vi "PArticle analysis.vi"() -> ()   [LabVIEW 2025]
uses:
  <vilib>/vision/NI_Vision_Development_Module.lvlib
panel:
  in  "White with color":bool
  out "Fail 2?":bool
  out "Fail 1?":bool
  out "Particle Reports (Pixels) 2":T1(array[cluster]) {"Orientation" format="%.2f"; "Dimensions"."Height" format="%.2f"; "Dimensions"."Width" format="%.2f"; "Center of Mass"."Y" format="%.2f"; "Center of Mass"."X" format="%.2f"; "Bounding Rect"."Bottom" format="%.2f"; "Bounding Rect"."Right" format="%.2f"; "Bounding Rect"."Top" format="%.2f"; "Bounding Rect"."Left" format="%.2f"; "Number of Holes" format="%.2f"; "Area" format="%.2f"}
  out "Particle Reports (Pixels)":T1(array[cluster]) {"Orientation" format="%.2f"; "Dimensions"."Height" format="%.2f"; "Dimensions"."Width" format="%.2f"; "Center of Mass"."Y" format="%.2f"; "Center of Mass"."X" format="%.2f"; "Bounding Rect"."Bottom" format="%.2f"; "Bounding Rect"."Right" format="%.2f"; "Bounding Rect"."Top" format="%.2f"; "Bounding Rect"."Left" format="%.2f"; "Number of Holes" format="%.2f"; "Area" format="%.2f"}
  out "Image 3":T2(plugin-control)
  out "Image 2":T2(plugin-control)
  out "Number of Particles 2":i32
  out "Number of Particles":i32
  out "Histogram Report 2":T3 {"Standard  Variation" format="%.2f"; "Mean Value" format="%.2f"; "Interval Width" format="%.2f"; "Starting Value" format="%.2f"; "Maximal Value" format="%.2f"; "Minimal Value" format="%.2f"}
  out "Image":T2(plugin-control)
  out "Histogram Report":T3 {"Standard  Variation" format="%.2f"; "Mean Value" format="%.2f"; "Interval Width" format="%.2f"; "Starting Value" format="%.2f"; "Maximal Value" format="%.2f"; "Minimal Value" format="%.2f"}
  in  "Interval Range":cluster{"Minimum":sgl, "Maximum":sgl} {"Maximum" format="%.2f"; "Minimum" format="%.2f"}
  # "1872"
  # "28883"
  # "31424"
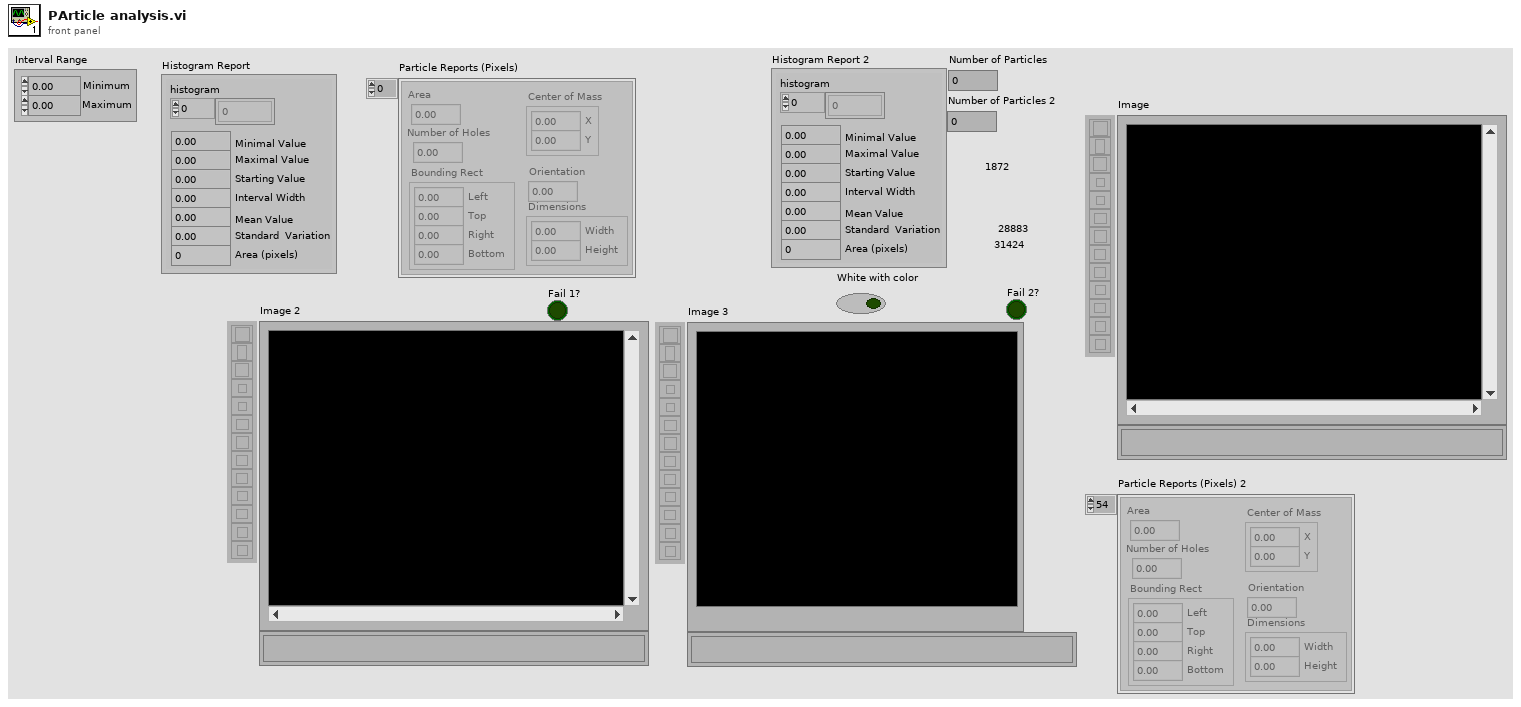
[diagram p1: front panel]
types:
  T1 = cluster{"Area":dbl, "Number of Holes":dbl, "Bounding Rect":cluster{"Left":dbl, "Top":dbl, "Right":dbl, "Bottom":dbl}, "Center of Mass":cluster{"X":dbl, "Y":dbl}, "Orientation":dbl, "Dimensions":cluster{"Width":dbl, "Height":dbl}}[]
  T2 = typedef "IMAQ Image.ctl" = refnum<image>
  T3 = cluster{"histogram":u32[], "Minimal Value":sgl, "Maximal Value":sgl, "Starting Value":sgl, "Interval Width":sgl, "Mean Value":sgl, "Standard  Variation":sgl, "Area (pixels)":i32}
  T4 = typedef "Image Type" = u32
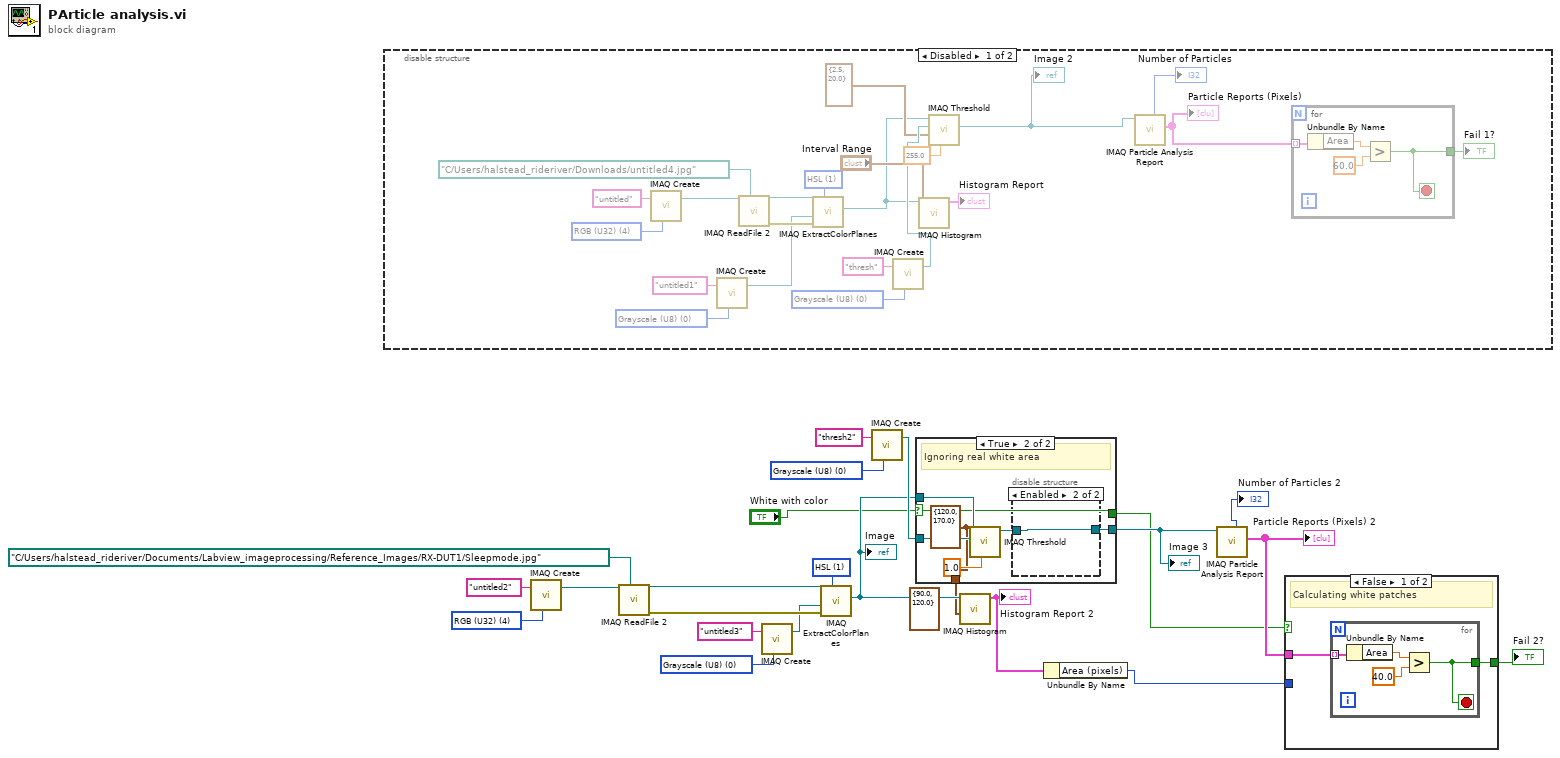
[diagram p0: block diagram]
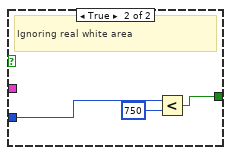
[diagram p3: hidden frame]
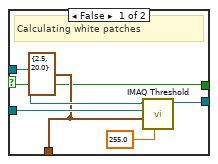
[diagram p4: hidden frame]
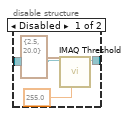
[diagram p5: hidden frame]
diagram:
  w13 = T4 0 items=["Grayscale (U8)", "Grayscale (I16)", "Grayscale (SGL)", "Complex (CSG)", "RGB (U32)", "HSL (U32)", "RGB (U64)", "Grayscale (U16)"] ("Image Type")
  (unwired) cluster{"Minimum":sgl, "Maximum":sgl} {"Minimum"=90.0, "Maximum"=120.0} ("Interval Range")
  w22 = u16 1 items=["RGB", "HSL", "HSV", "HSI"] ("Color Mode")
  w17 = T4 0 items=["Grayscale (U8)", "Grayscale (I16)", "Grayscale (SGL)", "Complex (CSG)", "RGB (U32)", "HSL (U32)", "RGB (U64)", "Grayscale (U16)"] ("Image Type")
  w16 = T4 4 items=["Grayscale (U8)", "Grayscale (I16)", "Grayscale (SGL)", "Complex (CSG)", "RGB (U32)", "HSL (U32)", "RGB (U64)", "Grayscale (U16)"] ("Image Type")
  n1 = disable-structure shown="Disabled" {
    frame Disabled {
      w33 = T4 0 items=["Grayscale (U8)", "Grayscale (I16)", "Grayscale (SGL)", "Complex (CSG)", "RGB (U32)", "HSL (U32)", "RGB (U64)", "Grayscale (U16)"] ("Image Type")
      w38 = u16 1 items=["RGB", "HSL", "HSV", "HSI"] ("Color Mode")
      w43 = T4 0 items=["Grayscale (U8)", "Grayscale (I16)", "Grayscale (SGL)", "Complex (CSG)", "RGB (U32)", "HSL (U32)", "RGB (U64)", "Grayscale (U16)"] ("Image Type")
      w44 = T4 4 items=["Grayscale (U8)", "Grayscale (I16)", "Grayscale (SGL)", "Complex (CSG)", "RGB (U32)", "HSL (U32)", "RGB (U64)", "Grayscale (U16)"] ("Image Type")
      n2 = call "IMAQ Create"("Image Name"="untitled", "Image Type"=w44) -> ("New Image"=w41:T2)  [unwired: 3 in, 1 out]
      n3 = call "IMAQ Create"("Image Name"="untitled1", "Image Type"=w43) -> ("New Image"=w30:T2)  [unwired: 3 in, 1 out]
      n4 = call "IMAQ ReadFile 2"("File Path"=path "C:/Users/halstead_rideriver/Downloads/untitled4.jpg", "Image"=w41) -> ("error out"=w39:errorcluster, "Image Out"=w37:T2)  [unwired: 5 in, 3 out]
      n5 = call "IMAQ ExtractColorPlanes"("Color Mode"=w38, "error in (no error)"=w39, "Green or Sat Plane"=w30, "Image Src"=w37) -> ("Green or Sat Plane out"=w29:T2)  [unwired: 4 in, 3 out]
      n6 = call "IMAQ Create"("Image Name"="thresh", "Image Type"=w33) -> ("New Image"=w32:T2)  [unwired: 3 in, 1 out]
      n7 = call "IMAQ Histogram"("Interval Range"="Interval Range", "Image"=w29) -> ("Histogram Report"=→"Histogram Report":T3)  [unwired: 8 in, 1 out]
      n8 = call "IMAQ Threshold"("Replace Value"=sgl 255.0, "Range"=cluster{"Lower value":sgl, "Upper value":sgl} {"Lower value"=2.5, "Upper value"=20.0}, "Image Dst"=w32, "Image Src"=w29) -> ("Image Dst Out"=w27:T2)  [unwired: 6 in, 1 out]
      "Image 2" <- w27
      n9 = call "IMAQ Particle Analysis Report"("Image"=w27) -> ("Particle Reports (Pixels)"=w25:T1, "Number of Particles"=→"Number of Particles":i32)  [unwired: 5 in, 4 out]
      "Particle Reports (Pixels)" <- w25
      n10 = for {
        tunnel: w25 -> [w49] mode=indexing
        tunnel: [w46] -> w26
        stop <- w46 stop-if-true
        n11 = Unbundle By Name(w49) -> ("Area"=w48:dbl)
        n12 = Greater?(x=w48, y=60.0) -> (0:w46:bool)
      }
      "Fail 1?" <- w26
    }
    frame Enabled {
    }
  }
  n13 = call "IMAQ Create"("Image Name"="untitled2", "Image Type"=w16) -> ("New Image"=w19:T2)  [unwired: 3 in, 1 out]
  n14 = call "IMAQ ReadFile 2"("File Path"=path "C:/Users/halstead_rideriver/Documents/Labview_imageprocessing/Reference_Images/RX-DUT1/Sleepmode.jpg", "Image"=w19) -> ("error out"=w21:errorcluster, "Image Out"=w23:T2)  [unwired: 5 in, 3 out]
  n15 = call "IMAQ Create"("Image Name"="untitled3", "Image Type"=w17) -> ("New Image"=w10:T2)  [unwired: 3 in, 1 out]
  n16 = call "IMAQ ExtractColorPlanes"("Color Mode"=w22, "error in (no error)"=w21, "Green or Sat Plane"=w10, "Image Src"=w23) -> ("Green or Sat Plane out"=w9:T2)  [unwired: 4 in, 3 out]
  "Image" <- w9
  n17 = call "IMAQ Create"("Image Name"="thresh2", "Image Type"=w13) -> ("New Image"=w11:T2)  [unwired: 3 in, 1 out]
  n18 = case shown="True" "White with color" {
    selector: "White with color" -> [w50 w56]
    tunnel: w11 -> [w53 w62]
    tunnel: w9 -> [w54 w61]
    tunnel: [w52 w59] -> w6
    tunnel: [w51 w57] -> w3
    tunnel: [w50 w56] -> w2
    frame False {
      w51 = cluster{"Lower value":sgl, "Upper value":sgl} {"Lower value"=2.5, "Upper value"=20.0} ("Range")
      # "Calculating white patches"
      n19 = call "IMAQ Threshold"("Replace Value"=sgl 255.0, "Range"=w51, "Image Dst"=w53, "Image Src"=w54) -> ("Image Dst Out"=w52:T2)  [unwired: 6 in, 1 out]
    }
    frame True {
      w57 = cluster{"Lower value":sgl, "Upper value":sgl} {"Lower value"=120.0, "Upper value"=170.0} ("Range")
      # "Ignoring real white area"
      n20 = call "IMAQ Threshold"("Replace Value"=sgl 1.0, "Range"=w57, "Image Dst"=w62, "Image Src"=w61) -> ("Image Dst Out"=w58:T2)  [unwired: 6 in, 1 out]
      n21 = disable-structure shown="Enabled" {
        disable-tunnel: [w64 w67] -> w59
        disable-tunnel: w58 -> [w63 w67]
        frame Disabled {
          n22 = call "IMAQ Threshold"("Replace Value"=sgl 255.0, "Range"=cluster{"Lower value":sgl, "Upper value":sgl} {"Lower value"=2.5, "Upper value"=20.0}, "Image Src"=w63) -> ("Image Dst Out"=w64:T2)  [unwired: 7 in, 1 out]
        }
        frame Enabled {
        }
      }
    }
  }
  "Image 3" <- w6
  n23 = call "IMAQ Histogram"("Interval Range"=w3, "Image"=w9) -> ("Histogram Report"=w14:T3)  [unwired: 8 in, 1 out]
  "Histogram Report 2" <- w14
  n24 = Unbundle By Name(w14) -> ("Area (pixels)"=w1:i32)
  n25 = call "IMAQ Particle Analysis Report"("Image"=w6) -> ("Particle Reports (Pixels)"=w8:T1, "Number of Particles"=→"Number of Particles 2":i32)  [unwired: 5 in, 4 out]
  "Particle Reports (Pixels) 2" <- w8
  n26 = case shown="False" w2 {
    tunnel: w8 -> [w69 _]
    tunnel: [w68 w74] -> w7
    tunnel: w1 -> [_ w76]
    frame False {
      # "Calculating white patches"
      n27 = for {
        tunnel: w69 -> [w73] mode=indexing
        tunnel: [w70] -> w68
        stop <- w70 stop-if-true
        n28 = Unbundle By Name(w73) -> ("Area"=w71:dbl)
        n29 = Greater?(x=w71, y=40.0) -> (0:w70:bool)
      }
    }
    frame True {
      # "Ignoring real white area"
      n30 = Less?(x=w76, y=750) -> (x < y?=w74:bool)
    }
  }
  "Fail 2?" <- w7
